vi "Write s4 acq config errors.vi"(8 "error in (no error)":errorcluster, 9 "acquisition config errors":T1, 10 "s4 acq config errors":T2, 11 "SPARC4_Channel in":refnum<class "SPARC4_Channel.lvclass">) -> (0 "error out":errorcluster, 3 "SPARC4_Channel out":refnum<class "SPARC4_Channel.lvclass">)   [LabVIEW 2018, in "SPARC4_Channel.lvclass"]
uses:
  SPARC4_Channel.lvclass
  SPARC4_Channel.lvclass/SPARC4_Channel.ctl
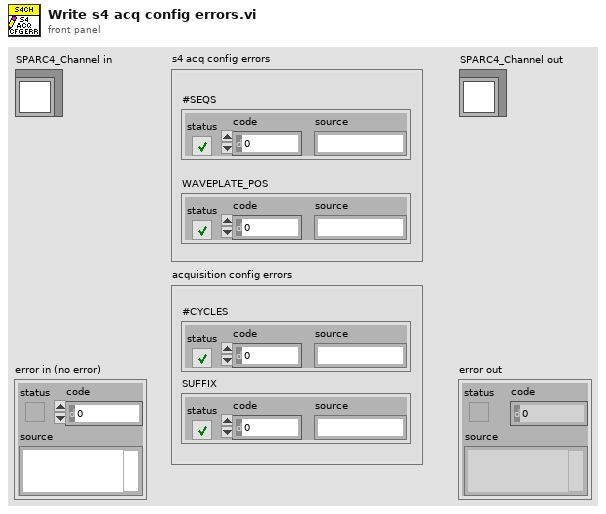
[diagram p1: front panel]
types:
  T1 = cluster{"#CYCLES":errorcluster, "SUFFIX":errorcluster}
  T2 = cluster{"#SEQS":errorcluster, "WAVEPLATE_POS":errorcluster}
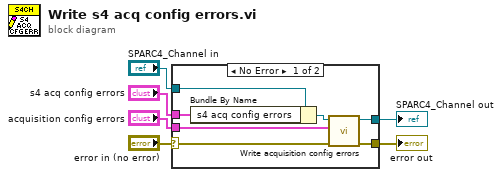
[diagram p0: block diagram]
diagram:
  n1 = case shown="No Error" "error in (no error)" {
    selector: "error in (no error)" -> [w9 w14]
    tunnel: [w10 w14] -> w5
    tunnel: [w11 w15] -> w3
    tunnel: "SPARC4_Channel in" -> [w13 w15]
    tunnel: "s4 acq config errors" -> [w8 _]
    tunnel: "acquisition config errors" -> [w7 _]
    frame No Error {
      n2 = Bundle By Name(cluster=w13, "s4 acq config errors"=w8) -> (w12:refnum<class "SPARC4_Channel.lvclass">)
      n3 = call-dynamic "Write acquisition config errors.vi"("error in (no error)"=w9, "acquisition config errors"=w7, "Channel in"=w12) -> ("error out"=w10:errorcluster, "Channel out"=w11:refnum<class "SPARC4_Channel.lvclass">)  [unwired: 7 in]
    }
    frame Error {
    }
  }
  "error out" <- w5
  "SPARC4_Channel out" <- w3
